vi "3. Pattern Matching.vi"() -> ()   [LabVIEW 2019]
doc: "c 2020 ReMiSYS All rights reserved."
panel:
  in  "Stop Button":bool
  out "Image Out":T1(plugin-control)
  # "c 2021 ReMiSYS All rights reserved."
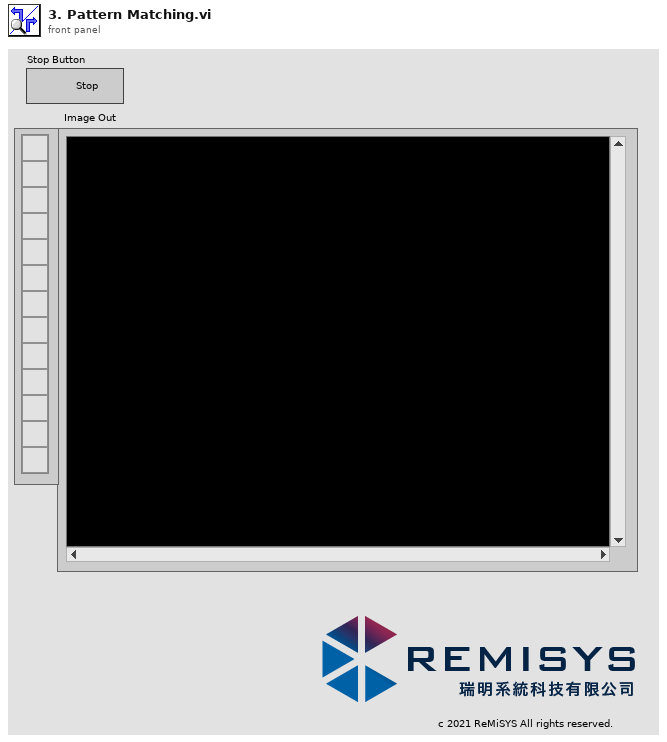
[diagram p1: front panel]
types:
  T1 = typedef "IMAQ Image.ctl" = refnum<image>
  T2 = typedef "Image Type" = u32
  T3 = cluster{"Desired Font (Application)":enum16{"User-specified Font", "Application Font", "System Font", "Dialog Font"}, "[User-specified Font]":cluster{"Font Name":string, "Size":i16, "Strikeout?":bool, "Italic?":bool, "Underline?":bool, "Outline?":bool, "Shadow?":bool, "Bold?":bool, "Rotation Angle":dbl}, "Horizontal Alignment":i16, "Vertical Alignment":i16}
  T4 = typedef "IMAQ GM Match Report.ctl" = cluster{"Position":cluster{"x":sgl, "y":sgl}, "Angle":sgl, "Scale":sgl, "Score":sgl, "Bounding Box":cluster{"x":sgl, "y":sgl}[], "Contrast Reversed":bool, "Occlusion %":sgl, "Template Target Curve Score":sgl, "Target Template Curve Score":sgl, "Correlation Score":sgl}
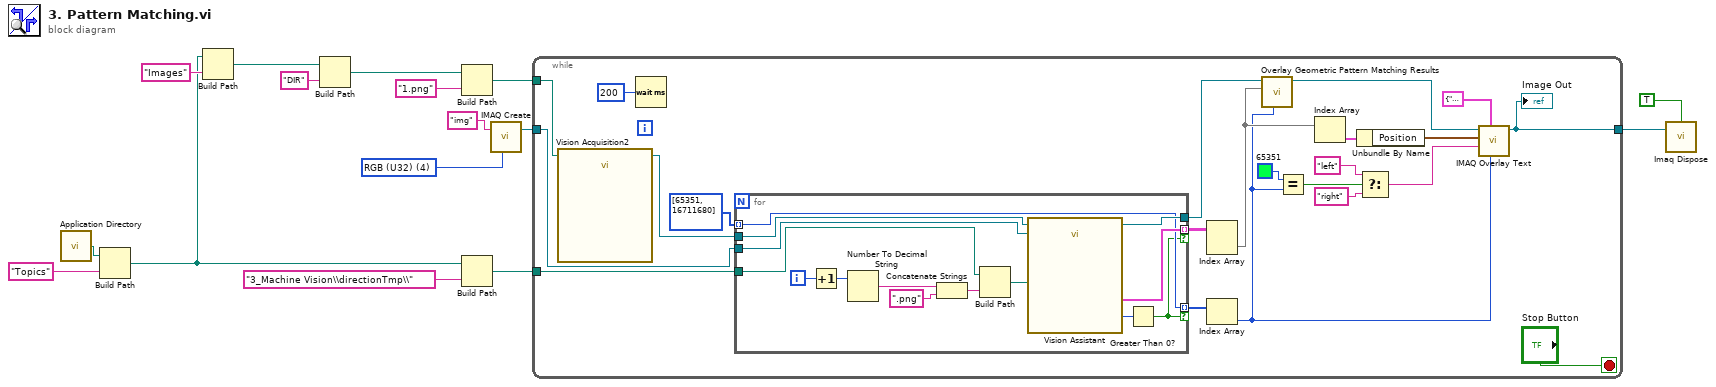
[diagram p0: block diagram]
diagram:
  w4 = T2 4 items=["Grayscale (U8)", "Grayscale (I16)", "Grayscale (SGL)", "Complex (CSG)", "RGB (U32)", "HSL (U32)", "RGB (U64)", "Grayscale (U16)"] ("Image Type")
  n1 = call <vilib>:"Application Directory.vi"() -> ("Application Directory"=w12:path)
  n2 = Build Path(base path=w12, name or relative path="Topics") -> (appended path=w6:path)
  n3 = Build Path(base path=w6, name or relative path="Images") -> (appended path=w8:path)
  n4 = Build Path(base path=w8, name or relative path="DIR") -> (appended path=w10:path)
  n5 = Build Path(base path=w10, name or relative path="1.png") -> (appended path=w9:path)
  n6 = Build Path(base path=w6, name or relative path="3_Machine Vision\\directionTmp\\") -> (appended path=w5:path)
  n7 = call "IMAQ Create"("Image Name"="img", "Image Type"=w4) -> ("New Image"=w2:T1)  [unwired: 3 in, 1 out]
  n8 = while {
    tunnel: w9 -> [w38]
    tunnel: w5 -> [w37]
    tunnel: w2 -> [w35]
    tunnel: [w27] -> w1
    stop <- "Stop Button" stop-if-true
    n9 = call "Vision Acquisition2"("Image Path"=w38) -> ("Image Out"=w36:T1)  [unwired: 2 in, 24 out]
    n10 = Wait (ms)(milliseconds to wait=u32 200) -> ()  [unwired: 1 out]
    n11 = for {
      tunnel: w37 -> [w48]
      tunnel: w36 -> [w45]
      tunnel: w35 -> [w39]
      tunnel: [w44] -> w31 mode=indexing if=w40
      tunnel: [w43] -> w33
      tunnel: [w42] -> w30 mode=indexing if=w40
      tunnel: u32[] [65351, 16711680] ("Color") -> [w42] mode=indexing
      i -> [w46]
      n12 = Increment(x=w46) -> (x+1=w49:i32)
      n13 = Number To Decimal String(number=w49) -> (decimal integer string=w52:string)  [unwired: 1 in]
      n14 = Concatenate Strings(w52, ".png" ("name or relative path")) -> (w50:string)
      n15 = Build Path(base path=w48, name or relative path=w50) -> (appended path=w47:path)
      n16 = call "Vision Assistant"("Image In"=w45, "Image Dst"=w39, "Template File Path (Pattern Matching 1)"=w47) -> ("Image Out"=w43:T1, "Matches (Pattern Matching 1)"=w44:T4[], "Number of Matches (Pattern Matching 1)"=w41:i32)  [unwired: 21 in, 1 out]
      n17 = Greater Than 0?(x=w41) -> (x > 0?=w40:bool)
    }
    n18 = Index Array(array=w31) -> (element=w26:T4[])  [unwired: 2 in]
    n19 = Index Array(array=w30) -> (element=w22:u32)  [unwired: 1 in]
    n20 = call "Overlay Geometric Pattern Matching Results.vi"("Color"=w22, "Matches"=w26, "Image"=w33) -> ("Image Out"=w28:T1)  [unwired: 2 in, 6 out]
    n21 = Equal?(x=u32 65351 ("Color"), y=w22) -> (x = y?=w21:bool)
    n22 = Index Array(array=w26) -> (element=w25:T4)  [unwired: 1 in]
    n23 = Unbundle By Name(w25) -> ("Position"=w24:cluster{"x":sgl, "y":sgl})
    n24 = Select(t="left" ("String"), s=w21, f="right") -> (s? t:f=w18:string)
    n25 = call "IMAQ Overlay Text"("Text Color (black)"=w22, "Font, Size & Style"=T3 {"Desired Font (Application)"=enum."User-specified Font", "[User-specified Font]"={"Font Name"="Arial", "Size"=40, "Strikeout?"=FALSE, "Italic?"=FALSE, "Underline?"=FALSE, "Outline?"=FALSE, "Shadow?"=FALSE, "Bold?"=FALSE, "Rotation Angle"=0.0}, "Horizontal Alignment"=1, "Vertical Alignment"=2}, "String"=w18, "Origin"=w24, "Image"=w28) -> ("Image Out"=w27:T1)  [unwired: 5 in, 1 out]
    "Image Out" <- w27
  }
  n26 = call "Imaq Dispose"("All Images? (No)"=TRUE, "Image"=w1) -> ()  [unwired: 4 in, 1 out]
